vi "LOC subReadWriteVIStringINIKeys(MulticolumnListbox).vi"(4 "Mode":enum16{"Read", "Write"}(ring), 5 "Section":string, 6 "error in (no error)":errorcluster, 8 "ConfigFileRefnum":T1, 9 "ControlRefnum":refnum<vi>) -> (0 "error out":errorcluster)   [LabVIEW 2020, in "Localization_Tools.lvlib"]
uses:
  Localization_Tools.lvlib
  <vilib>/Utility/config.llb/Config Data RefNum.ctl
  <vilib>/Utility/config.llb/NI_LVConfig.lvlib
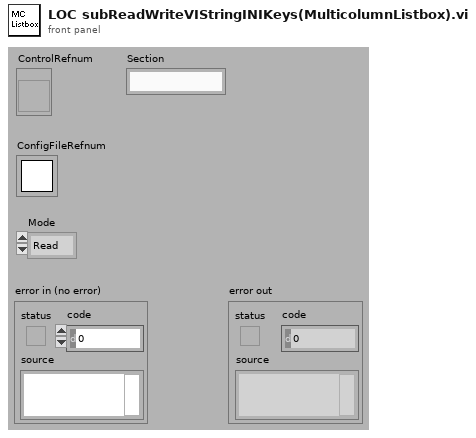
[diagram p1: front panel]
types:
  T1 = typedef "NI_LVConfig.lvlib/Config Data RefNum.ctl" = refnum<k1>
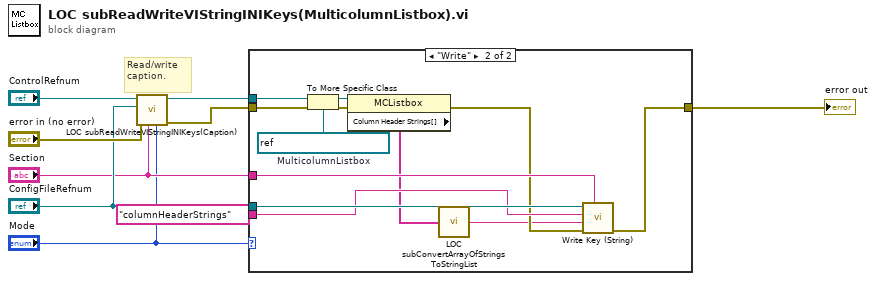
[diagram p0: block diagram]
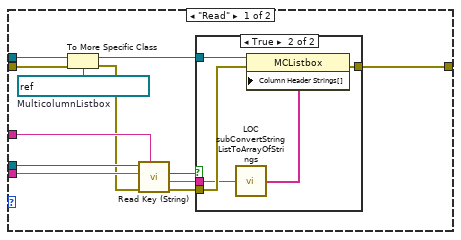
[diagram p2: hidden frame]
diagram:
  # "Read/write\ncaption."
  n1 = call "LOC subReadWriteVIStringINIKeys(Caption).vi"("Mode"="Mode", "Section"="Section", "error in (no error)"="error in (no error)", "ConfigFileRefnum"="ConfigFileRefnum", "ControlRefnum"="ControlRefnum") -> ("error out"=w5:errorcluster, "dup ControlRefnum"=w7:refnum<vi>)  [unwired: 3 in]
  n2 = case shown="\"Write\"" "Mode" {
    tunnel: w7 -> [w17 w38]
    tunnel: w5 -> [w16 w37]
    tunnel: "ConfigFileRefnum" -> [w21 w34]
    tunnel: "Section" -> [w20 w32]
    tunnel: "columnHeaderStrings" ("key") -> [w19 w33]
    tunnel: [w12 w30] -> w1
    frame "Read" {
      w18 = refnum<vi> refnum  # MulticolumnListbox
      n3 = To More Specific Class(target class=w18, reference=w17, error in=w16) -> (specific class reference=w14:refnum<vi>, error out=w15:errorcluster)
      n4 = call <vilib>:"Read Key (String).vi"("section"=w20, "error in (no error)"=w15, "key"=w19, "refnum"=w21) -> ("error out"=w13:errorcluster, "value"=w11:string, "found?"=w10:bool)  [unwired: 4 in, 1 out]
      n5 = case shown="True" w10 {
        tunnel: w14 -> [_ w27]
        tunnel: w13 -> [w22 w26]
        tunnel: [w22 w25] -> w12
        tunnel: w11 -> [_ w24]
        frame False {
        }
        frame True {
          n6 = call "LOC subConvertStringListToArrayOfStrings.vi"("InputString"=w24) -> ("OutputArray"=w23:string[])
          n7 = property class="MCListbox"(reference=w27, error in=w26, "Column Header Strings[]"=w23) -> (error out=w25:errorcluster)  [unwired: 1 out]
        }
      }
    }
    frame "Write" {
      w39 = refnum<vi> refnum  # MulticolumnListbox
      n8 = To More Specific Class(target class=w39, reference=w38, error in=w37) -> (specific class reference=w36:refnum<vi>, error out=w35:errorcluster)
      n9 = property class="MCListbox"(reference=w36, error in=w35) -> (error out=w31:errorcluster, "Column Header Strings[]"=w29:string[])  [unwired: 1 out]
      n10 = call "LOC subConvertArrayOfStringsToStringList.vi"("InputArray"=w29) -> ("OutputString"=w28:string)
      n11 = call <vilib>:"Write Key (String).vi"("section"=w32, "error in (no error)"=w31, "value"=w28, "key"=w33, "refnum"=w34) -> ("error out"=w30:errorcluster)  [unwired: 4 in, 2 out]
    }
  }
  "error out" <- w1
